vi "Post-Build Custom Action.vi"() -> (0 "error out":errorcluster)   [LabVIEW 2020]
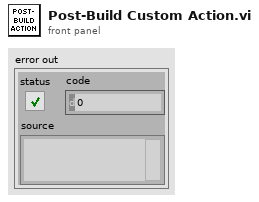
[diagram p1: front panel]
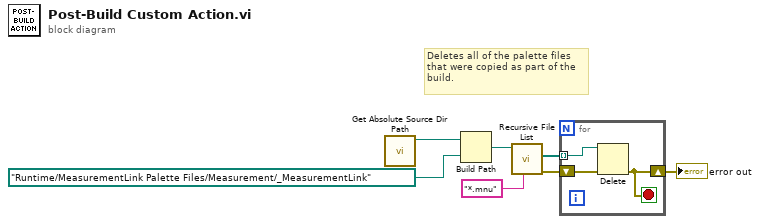
[diagram p0: block diagram]
diagram:
  # "Deletes all of the palette files\nthat were copied as part of the\nbuild."
  n1 = call "Get Absolute Source Dir Path.vi"() -> ("source dir"=w1:path)  [unwired: 11 in]
  n2 = Build Path(base path=w1, name or relative path=path "Runtime/MeasurementLink Palette Files/Measurement/_MeasurementLink") -> (appended path=w2:path)
  n3 = call <vilib>:"Recursive File List.vi"("pattern"="*.mnu", "Folder Path"=w2) -> ("error out"=w5:errorcluster, "All Files in Dir"=w6:path[])  [unwired: 5 in, 3 out]
  n4 = for {
    tunnel: w6 -> [w10] mode=indexing
    shift-right: [w8] -> w3
    shift-left: w5 -> [w9]
    stop <- w8 stop-if-true
    n5 = Delete(path (use dialog)=w10, error in=w9) -> (error out=w8:errorcluster)  [unwired: 3 in, 2 out]
  }
  "error out" <- w3
